vi "DACreadglobal.vi"() -> ()   [LabVIEW 2011]
panel:
  out "DAC read global (mV)":dbl[](array[numeric])
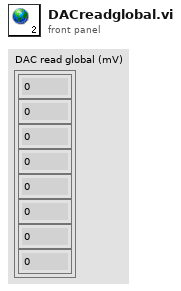
[diagram p1: front panel]
diagram:
